vi "FG VFH Parameters.vi"(2 "FG Action (Read)":T3, 3 "VFH Parameters in":T1={"Robot Radius"=100, "Near Threshold"=100, "Mid Threshold"=200, "Far Threshold"=300, "Weights"={"TS-S weight"=90.0, "CS-S weight"=90.0, "PCS-S weight"=90.0, "Near weight"=90.0, "Mid weight"=90.0, "Far weight"=90.0}}) -> (1 "VFH Parameters out":T1={"Robot Radius"=100, "Near Threshold"=100, "Mid Threshold"=200, "Far Threshold"=300, "Weights"={"TS-S weight"=90.0, "CS-S weight"=90.0, "PCS-S weight"=90.0, "Near weight"=90.0, "Mid weight"=90.0, "Far weight"=90.0}})   [LabVIEW 2009]
uses:
  Actions for FG's.ctl
  Intelligence/VFH/VFH Parameters.ctl
  Intelligence/VFH/VFH Weights.ctl
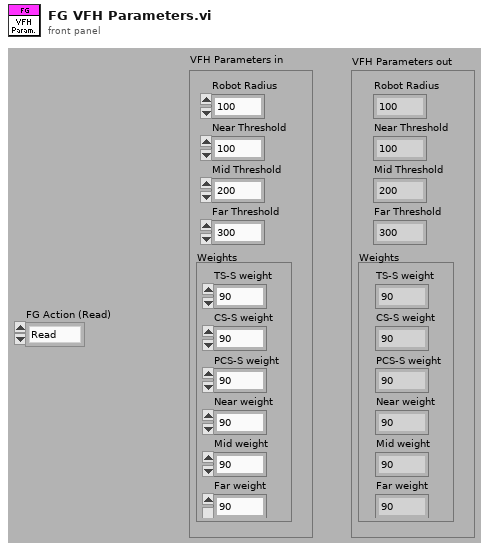
[diagram p1: front panel]
types:
  T1 = typedef "VFH Parameters.ctl" = cluster{"Robot Radius":u16, "Near Threshold":u16, "Mid Threshold":u16, "Far Threshold":u16, "Weights":T2}
  T2 = typedef "VFH Weights.ctl" = cluster{"TS-S weight":dbl, "CS-S weight":dbl, "PCS-S weight":dbl, "Near weight":dbl, "Mid weight":dbl, "Far weight":dbl}
  T3 = typedef "Actions for FG's.ctl" = enum16{"Read", "Write"}
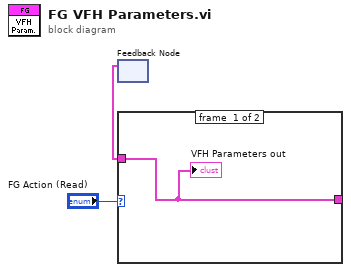
[diagram p0: block diagram]
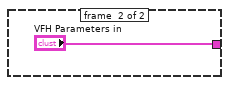
[diagram p2: hidden frame]
diagram:
  n1 = feedback #1() -> (w3:T1)  [unwired: 1 in]
  n2 = case shown="\"Read\", Default" "FG Action (Read)" {
    tunnel: [w4 "VFH Parameters in"] -> w2
    tunnel: w3 -> [w4 _]
    frame #0 {
      "VFH Parameters out" <- w4
    }
    frame #1 {
    }
  }
